vi "initAsyncJob.vi"(8 "error in (no error)":errorcluster, 11 "Job in":refnum<class "Job.lvclass">) -> (0 "error out":errorcluster, 3 "Job out":refnum<class "Job.lvclass">)   [LabVIEW 2013, in "openCronJob.lvlib" / "Job.lvclass"]
uses:
  Job.lvclass
  Job.lvclass/Job.ctl
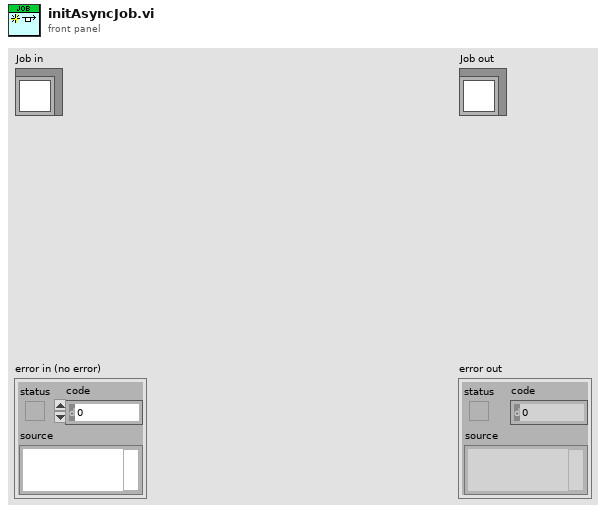
[diagram p1: front panel]
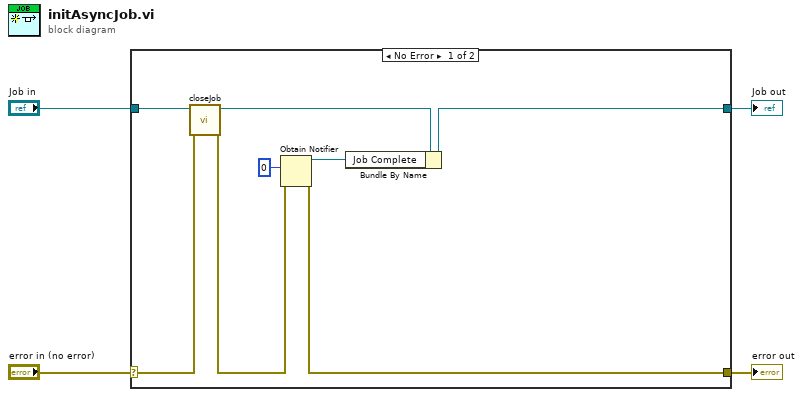
[diagram p0: block diagram]
diagram:
  n1 = case shown="No Error" "error in (no error)" {
    selector: "error in (no error)" -> [w6 w14]
    tunnel: [w9 w14] -> w3
    tunnel: [w10 w13] -> w1
    tunnel: "Job in" -> [w8 w13]
    frame No Error {
      n2 = call "closeJob.vi"("error in (no error)"=w6, "Job in"=w8) -> ("error out"=w5:errorcluster, "Job out"=w7:refnum<class "Job.lvclass">)  [unwired: 8 in]
      n3 = Obtain Notifier(notification data type=0 ("exception"), error in (no error)=w5) -> (notifier out=w11:refnum<notifier>, error out=w9:errorcluster)  [unwired: 2 in, 1 out]
      n4 = Bundle By Name(cluster=w7, "Job Complete"=w11) -> (w10:refnum<class "Job.lvclass">)
    }
    frame Error {
    }
  }
  "error out" <- w3
  "Job out" <- w1
